vi "Arduino_FindPaths.vi"(8 "error in (no error)":errorcluster, 11 "Arduino In":T1={"Java"=path "/Applications/Arduino.app/Contents/Java", "Packages"=path "/Users/crogers/Library/Arduino15/packages", "folder"=path "", "serial"="", "Console"=""}) -> (0 "error out":errorcluster, 1 "temp code file":path, 2 "Name":string="Code", 3 "Arduino In out":T1)   [LabVIEW 2020]
uses:
  Arduino.ctl
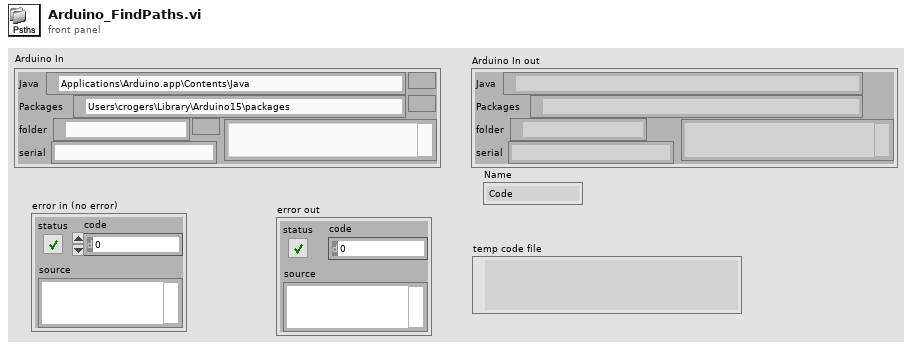
[diagram p1: front panel]
types:
  T1 = typedef "Arduino.ctl" = cluster{"Java":path, "Packages":path, "folder":path, "serial":string, "Console":string}
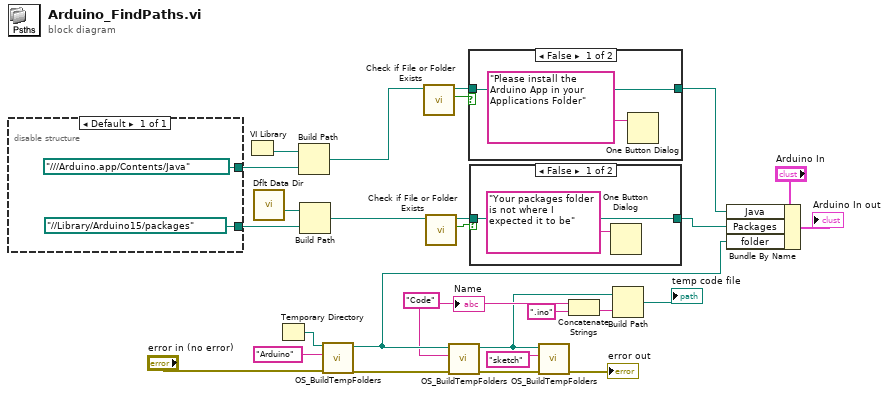
[diagram p0: block diagram]
diagram:
  w13 = "Code" ("Name")
  n1 = disable-structure shown="Default" {
    disable-tunnel: [path "../../../Arduino.app/Contents/Java"] -> w24
    disable-tunnel: [path "../../Library/Arduino15/packages"] -> w23
    frame Enabled {
    }
  }
  n2 = VI Library() -> (path=w25:path)
  n3 = call <vilib>:"Dflt Data Dir.vi"() -> ("App:Default Data Directory"=w22:path)
  n4 = Temporary Directory() -> (w20:path)
  n5 = Build Path(base path=w25, name or relative path=w24) -> (appended path=w6:path)
  n6 = Build Path(base path=w22, name or relative path=w23) -> (appended path=w5:path)
  n7 = call "OS_BuildTempFolders.vi"("error in (no error)"="error in (no error)", "name"="Arduino" ("name or relative path"), "path"=w20) -> ("error out"=w9:errorcluster, "appended path"=w16:path)  [unwired: 7 in]
  n8 = call <vilib>:"Check if File or Folder Exists.vi"("path"=w6) -> ("file or folder exists?"=w21:bool, "dup path"=w1:path)  [unwired: 8 in, 1 out]
  n9 = call <vilib>:"Check if File or Folder Exists.vi"("path"=w5) -> ("file or folder exists?"=w7:bool, "dup path"=w4:path)  [unwired: 8 in, 1 out]
  n10 = call "OS_BuildTempFolders.vi"("error in (no error)"=w9, "name"=w13, "path"=w16) -> ("error out"=w17:errorcluster, "appended path"=w11:path)  [unwired: 7 in]
  n11 = case shown="False" w21 {
    tunnel: [w30 w32] -> w2
    tunnel: w1 -> [w30 w32]
    frame False {
      n12 = One Button Dialog(message="Please install the Arduino App in your Applications Folder") -> ()  [unwired: 1 in, 1 out]
    }
    frame True {
    }
  }
  n13 = case shown="False" w7 {
    tunnel: [w33 w35] -> w3
    tunnel: w4 -> [w33 w35]
    frame False {
      n14 = One Button Dialog(message="Your packages folder is not where I expected it to be") -> ()  [unwired: 1 in, 1 out]
    }
    frame True {
    }
  }
  n15 = call "OS_BuildTempFolders.vi"("error in (no error)"=w17, "name"="sketch" ("name or relative path"), "path"=w11) -> ("error out"=→"error out":errorcluster)  [unwired: 7 in, 1 out]
  n16 = Concatenate Strings(w13, ".ino" ("string")) -> (w14:string)
  n17 = Build Path(base path=w11, name or relative path=w14) -> (appended path=→"temp code file":path)
  n18 = Bundle By Name(cluster="Arduino In", "Java"=w2, "Packages"=w3, "folder"=w16) -> (→"Arduino In out":T1)
  "Name" <- w13
